vi "FGV_logger.vi"(8 "error in":errorcluster, 9 "?":T1={"Column"=-1, "Data"=""}, 11 "Command":enum16{"Update", "Log", "Init"}(ring)) -> (0 "error out":errorcluster)   [LabVIEW 2016]
uses:
  Typedef/LogInput.ctl
  <vilib>/Utility/file.llb/Write Delimited Spreadsheet (string).vi
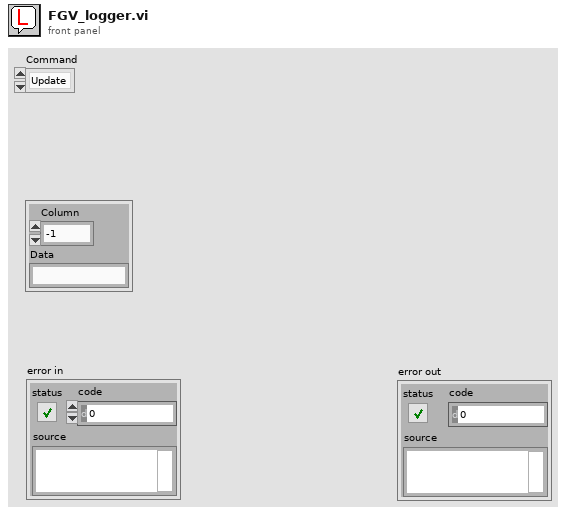
[diagram p1: front panel]
types:
  T1 = typedef "LogInput.ctl" = cluster{"Column":i32, "Data":string}
  T2 = enum16{"open", "replace", "create", "open or create", "replace or create", "replace or create with confirmation"}
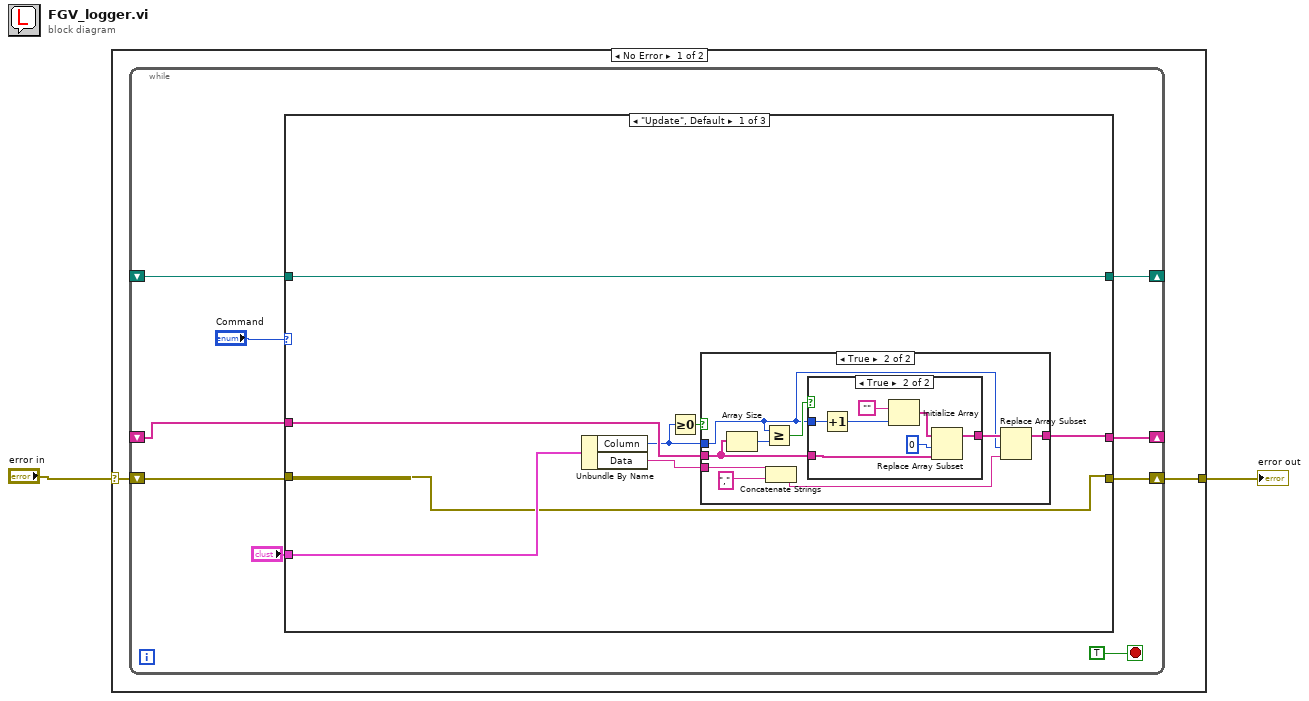
[diagram p0: block diagram]
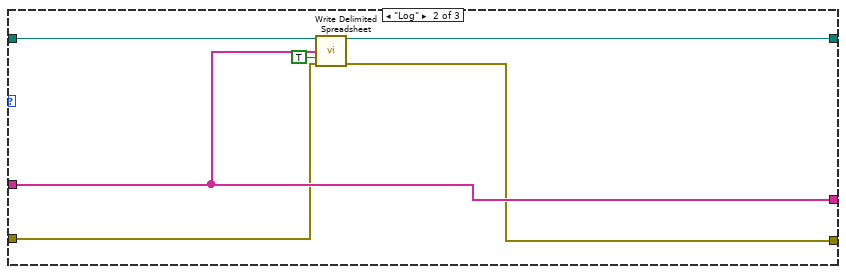
[diagram p4: hidden frame]
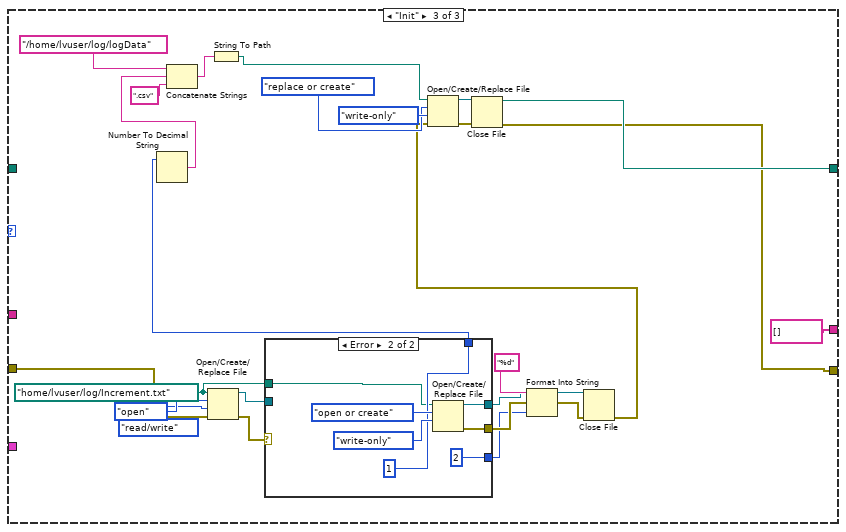
[diagram p5: hidden frame]
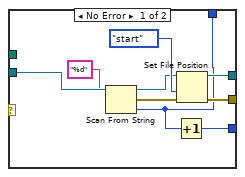
[diagram p6: hidden frame]
diagram:
  n1 = case shown="No Error" "error in" {
    selector: "error in" -> [w4 w88]
    tunnel: [w3 w88] -> w1
    frame No Error {
      n2 = while {
        shift-right: [w10] -> _
        shift-left: _ -> [w9]
        shift-right: [w7] -> w3
        shift-left: w4 -> [w8]
        shift-right: [w6] -> _
        shift-left: _ -> [w5]
        stop <- TRUE stop-if-true
        n3 = case shown="\"Update\", Default" "Command" {
          tunnel: "?" -> [w21 _ _]
          tunnel: [w18 w45 string[] []] -> w10
          tunnel: w9 -> [w20 w45 _]
          tunnel: w8 -> [w17 w41 w66]
          tunnel: [w17 w40 w50] -> w7
          tunnel: [w14 w44 w51] -> w6
          tunnel: w5 -> [w14 w43 _]
          frame "Update", Default {
            n4 = Unbundle By Name(w21) -> ("Column"=w15:i32, "Data"=w19:string)
            n5 = Greater Or Equal To 0?(x=w15) -> (x >= 0?=w16:bool)
            n6 = case shown="True" w16 {
              tunnel: w20 -> [w22 w29]
              tunnel: w19 -> [_ w23]
              tunnel: [w22 w27] -> w18
              tunnel: w15 -> [_ w26]
              frame False {
              }
              frame True {
                n7 = Array Size(array=w29) -> (size(s)=w31:i32)
                n8 = Greater Or Equal?(x=w26, y=w31) -> (x >= y?=w30:bool)
                n9 = Concatenate Strings(w23, ",") -> (w25:string)
                n10 = case shown="True" w30 {
                  tunnel: w29 -> [w32 w35]
                  tunnel: [w32 w34] -> w28
                  tunnel: w26 -> [_ w38]
                  frame False {
                  }
                  frame True {
                    n11 = Increment(x=w38) -> (x+1=w33:i32)
                    n12 = Initialize Array("", w33) -> (w37:string[])
                    n13 = Replace Array Subset(array=w37, new element=w35, index=0) -> (w34:string[])
                  }
                }
                n14 = Replace Array Subset(array=w28, new element=w25, index=w26) -> (w27:string[])
              }
            }
          }
          frame "Log" {
            n15 = call-poly <vilib>:"Write Delimited Spreadsheet.vi"("file path (dialog if empty)"=w43, "1D data"=w45, "append to file? (new file:F)"=TRUE, "error in (no error)"=w41) -> ("new file path (Not A Path if cancelled)"=w44:path, "error out"=w40:errorcluster)  [unwired: 10 in]
          }
          frame "Init" {
            w46 = path "/home/lvuser/log/Increment.txt" ("file path (use dialog)")
            n16 = Open/Create/Replace File(file path (use dialog)=w46, error in=w66, operation (0:open)=T2."open", access (0:read/write)=enum16{"read/write", "read-only", "write-only"}."read/write") -> (refnum out=w65:refnum<file>, error out=w47:errorcluster)  [unwired: 2 in, 1 out]
            n17 = case shown="Error" w47 {
              tunnel: w65 -> [w80 _]
              tunnel: [w76 w82] -> w63
              tunnel: [w75 w83] -> w62
              tunnel: [w73 2] -> w61
              tunnel: [w72 1] -> w55
              tunnel: w46 -> [_ w81]
              frame No Error {
                n18 = Scan From String("%d" ("format string"), w80) -> (w77:refnum<file>, w74:errorcluster, output 1=w72:i32)  [unwired: 2 in]
                n19 = Increment(x=w72) -> (x+1=w73:i32)
                n20 = Set File Position(refnum=w77, from (0:start)=enum16{"start", "end", "current"}."start", error in=w74) -> (refnum out=w76:refnum<file>, error out=w75:errorcluster)  [unwired: 1 in]
              }
              frame Error {
                n21 = Open/Create/Replace File(file path (use dialog)=w81, operation (0:open)=T2."open or create", access (0:read/write)=enum16{"read/write", "read-only", "write-only"}."write-only") -> (refnum out=w82:refnum<file>, error out=w83:errorcluster)  [unwired: 3 in, 1 out]
              }
            }
            n22 = Number To Decimal String(number=w55) -> (decimal integer string=w54:string)  [unwired: 1 in]
            n23 = Concatenate Strings("/home/lvuser/log/logData" ("string"), w54, ".csv" ("string")) -> (w57:string)
            n24 = String To Path(string=w57) -> (path=w56:path)
            n25 = Format Into String(format string="%d", initial string=w63, error in=w62, w61) -> (resulting string=w60:refnum<file>, error out=w59:errorcluster)
            n26 = Close File(refnum=w60, error in=w59) -> (error out=w58:errorcluster)  [unwired: 1 out]
            n27 = Open/Create/Replace File(file path (use dialog)=w56, error in=w58, operation (0:open)=T2."replace or create", access (0:read/write)=enum16{"read/write", "read-only", "write-only"}."write-only") -> (refnum out=w52:refnum<file>, error out=w53:errorcluster)  [unwired: 2 in, 1 out]
            n28 = Close File(refnum=w52, error in=w53) -> (path=w51:path, error out=w50:errorcluster)
          }
        }
      }
    }
    frame Error {
    }
  }
  "error out" <- w1
